vi "Update Online List.vi"(8 "error in (no error)":errorcluster, 10 "Online Users":string[](array[string]), 11 "Chat Window Model in":refnum<class "Chat Window Model.lvclass">) -> (0 "error out":errorcluster, 3 "Chat Window Model out":refnum<class "Chat Window Model.lvclass">)   [LabVIEW 2019, in "Chat Window Model.lvlib" / "Chat Window Model.lvclass"]
uses:
  Chat Window Model.lvclass
  Chat Window Model.lvclass/Chat Window Model.ctl
  Chat Window UI Controller/Chat Window UI Controller Messages/Update Online List Msg/Update Online List Msg.lvclass/Update Online List Msg.ctl
  <vilib>/ActorFramework/Message Enqueuer/Message Enqueuer.lvclass/Message Enqueuer.ctl
  <vilib>/ActorFramework/Message Enqueuer/Enqueue.vi
  Chat Window UI Controller/Chat Window UI Controller Messages/Update Online List Msg/Update Online List Msg.lvclass
  C:/Program Files/National Instruments/LabVIEW 2019/vi.lib/ActorFramework/Message/Message.lvclass
  <vilib>/ActorFramework/Message Priority Queue/Priority Enqueue.vi
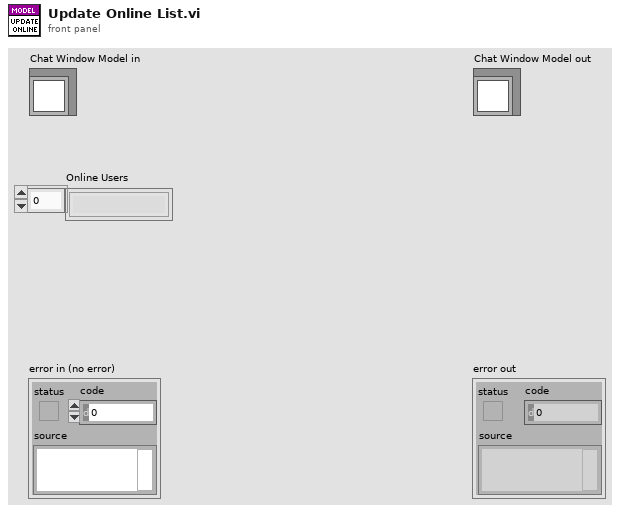
[diagram p1: front panel]
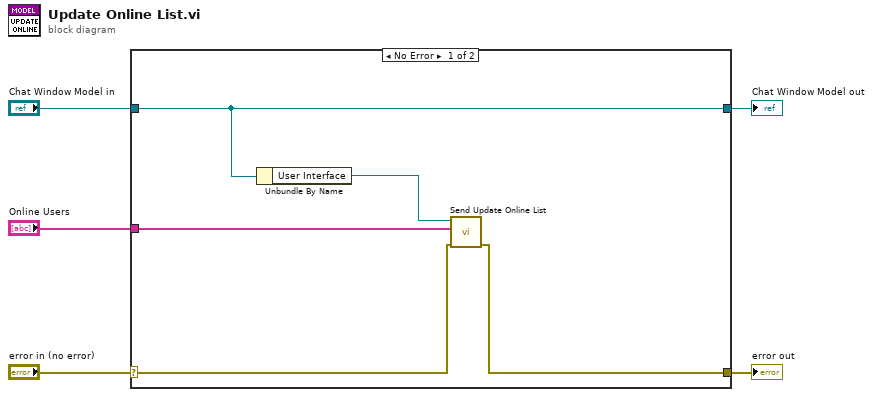
[diagram p0: block diagram]
diagram:
  n1 = case shown="No Error" "error in (no error)" {
    selector: "error in (no error)" -> [w7 w12]
    tunnel: [w6 w12] -> w4
    tunnel: [w10 w11] -> w2
    tunnel: "Chat Window Model in" -> [w10 w11]
    tunnel: "Online Users" -> [w8 _]
    frame No Error {
      n2 = Unbundle By Name(w10) -> ("User Interface"=w9:refnum<class "Message Enqueuer.lvclass">)
      n3 = call "Send Update Online List.vi"("error in (no error)"=w7, "Online List"=w8, "Message Enqueuer"=w9) -> ("error out"=w6:errorcluster)  [unwired: 7 in, 1 out]
    }
    frame Error {
    }
  }
  "error out" <- w4
  "Chat Window Model out" <- w2
